vi "fpga_status.vi"(8 "error in (no error)":errorcluster, 11 "p2p vst in":refnum<class "p2p vst.lvclass">) -> (0 "error out":errorcluster, 2 "pulse TX status":T1, 3 "p2p vst out":refnum<class "p2p vst.lvclass">)   [LabVIEW 2021, in "p2p vst.lvclass"]
uses:
  p2p vst.lvclass
  p2p vst.lvclass/p2p vst.ctl
  <vilib>/rvi/interface/nirviReadWriteControl/nirviReadWriteControl.xnode
  NiFpgaLv.dll
  <vilib>/Utility/error.llb/Error Cluster From Error Code.vi
  <vilib>/rvi/interface/Simulation/niFpgaSimulationCallBeginRW.vi
  <vilib>/rvi/errors/niLvFpgaAdjustHostInterfaceError.vi
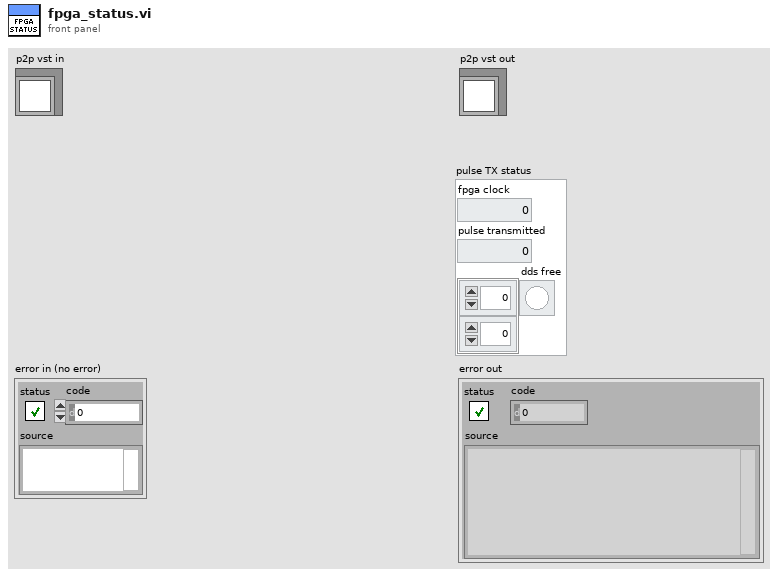
[diagram p1: front panel]
types:
  T1 = cluster{"fpga clock":dbl, "pulse transmitted":u32, "dds free":bool[][]}
  T2 = cluster{"fpga clock":u64, "pulse transmitted":u32, "dds free":bool[]}
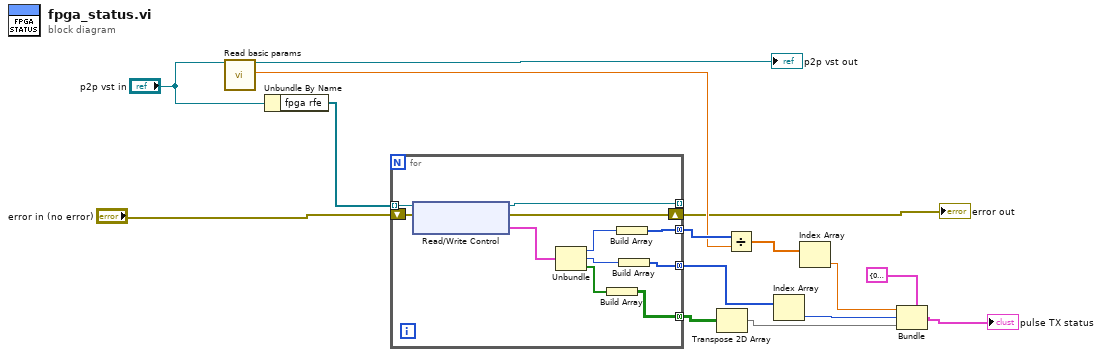
[diagram p0: block diagram]
diagram:
  n1 = call-dynamic "Read basic params.vi"("device_type in"="p2p vst in") -> ("device_type out"=→"p2p vst out":refnum<class "p2p vst.lvclass">, "Fs  FPGA"=w12:dbl)  [unwired: 13 in, 4 out]
  n2 = Unbundle By Name("p2p vst in") -> ("fpga rfe"=w14:refnum<k20>[])
  n3 = for {
    tunnel: w14 -> [w23] mode=indexing
    shift-right: [w25] -> w2
    shift-left: "error in (no error)" -> [w26]
    tunnel: [w24] -> _ mode=indexing
    tunnel: [w22] -> w13 mode=concatenating
    tunnel: [w21] -> w8 mode=concatenating
    tunnel: [w20] -> w15 mode=concatenating
    n4 = xnode "Read/Write Control"("FPGA VI Reference In"=w23, "error in"=w26) -> ("FPGA VI Reference Out"=w24:refnum<k20>, "error out"=w25:errorcluster, "pulse TX status"=w19:T2)
    n5 = Unbundle(w19) -> ("fpga clock"=w18:u64, "pulse transmitted"=w17:u32, "dds free"=w16:bool[])
    n6 = Build Array(w16) -> (w22:bool[][])
    n7 = Build Array(w18) -> (w20:u64[])
    n8 = Build Array(w17) -> (w21:u32[])
  }
  "error out" <- w2
  n9 = Transpose 2D Array(2D array=w13) -> (transposed array=w11:bool[][])
  n10 = Divide(x=w15, y=w12) -> (x/y=w10:dbl[])
  n11 = Index Array(array=w8) -> (element=w7:u32)  [unwired: 1 in]
  n12 = Index Array(array=w10) -> (element=w9:dbl)  [unwired: 1 in]
  n13 = Bundle(cluster=T1 {"fpga clock"=0.0, "pulse transmitted"=0, "dds free"=[[FALSE, FALSE, FALSE, FALSE, FALSE, FALSE, FALSE, FALSE, FALSE, FALSE, FALSE, FALSE, FALSE, FALSE, FALSE, FALSE]]} ("pulse TX status"), "fpga clock"=w9, "pulse transmitted"=w7, "dds free"=w11) -> (→"pulse TX status":T1)
